vi "Write Packet Buffer.vi"(0 "data fifo in":refnum<k21>, 1 "reset":bool, 5 "sizes fifo in":refnum<k21>, 7 "serialized data":u8[](array[numeric])=[0, 0, 0, 0, 0, 0, 0, 0], 9 "input valid":bool, 11 "valid bytes in":fxp<+,4,4>, 12 "end of packet":bool) -> (4 "data fifo out":refnum<k21>, 6 "sizes fifo out":refnum<k21>, 14 "ready for input":bool)   [LabVIEW 2020, in "GettingStarted_Acq_Tap_148X_FPGA.lvlib"]
uses:
  <instrlib>/_niInstr/Data Formatting/v1/FPGA/Private/Convert/U8 array to Boolean Array.vi
  <vilib>/rvi/DataTransferAndStorage/Container/Common/niFpgaContainerExecOnDevCompGetState.vi
  <vilib>/rvi/Emulation/niFpgaEmulationIsFPGAContextNoSignature.vi
  <vilib>/rvi/Emulation/niFpgaSctlEmulationGetInTimedLoop.vi
  <vilib>/rvi/errors/niFpgaSetErrorForExecOnDevCompSimple.vi
  <vilib>/rvi/eio/common/nirviEmuReportErrorAndStop.vi
  <vilib>/rvi/DataTransferAndStorage/Container/Common/niFpgaContainerGetUniqueNameForEmu.vi
  <vilib>/rvi/FIFO/Fifo_Resource/nirvififoEmulationSetSize.vi
  <vilib>/rvi/FIFO/Fifo_Resource/nirviFifoEmulationQueueMgr.vi
  <instcachedir>/0/nirviFifoEmulationQueueMgr_E5CAEC123FF24DC58D834DCA3CDAA9B5.lvgen/nirviFifoEmulationQueueMgr_E5CAEC123FF24DC58D834DCA3CDAA9B5_000.vi
  <vilib>/rvi/FIFO/Fifo_Resource/nirvififoEmulationDetermineInputValidOut.vi
  <vilib>/rvi/FIFO/Fifo_Resource/nirvififoEmulationCreateLock.vi
  <vilib>/rvi/Emulation/niFpgaProcessEmulError.vi
  <vilib>/rvi/FIFO/Fifo_Resource/nirvififoEmulationObtainLock.vi
  <vilib>/rvi/FIFO/Fifo_Resource/nirvififoEmulationReleaseLock.vi
  <vilib>/rvi/occurrence/nirviWaitOnOccurrenceBase.vi
  <vilib>/rvi/errors/nirviReportUnexpectedCaseInternalError.vi
  <vilib>/rvi/errors/nirviReportUnexpectedCaseInternalError (U32).vi
  <vilib>/Utility/error.llb/Clear Errors.vi
  <vilib>/rvi/interface/RandomDataEmulation/niFpgaRandomDataHandleErrors.vi
  <instcachedir>/0/nirviFifoEmulationQueueMgr_E5CAEC123FF24DC58D834DCA3CDAA9B5.lvgen/nirviFifoEmulationQueueMgr_E5CAEC123FF24DC58D834DCA3CDAA9B5_012.vi
  <vilib>/rvi/DataTransferAndStorage/Container/XNode/niFpgaContainer.xnode
  <vilib>/rvi/FIFO/Fifo_Resource/niFpgaFifoEmulationRefIn.vi
  GettingStarted_Acq_Tap_148X_FPGA.lvlib
  <instrlib>/_niInstr/Data Formatting/v1/FPGA/niInstr Data Formatting v1 FPGA.lvlib
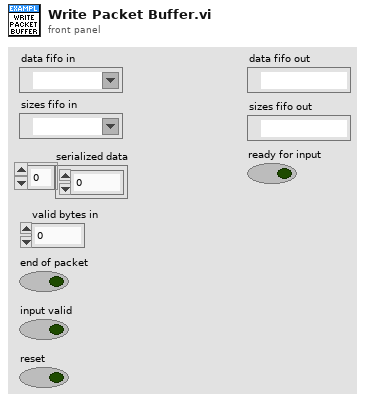
[diagram p1: front panel]
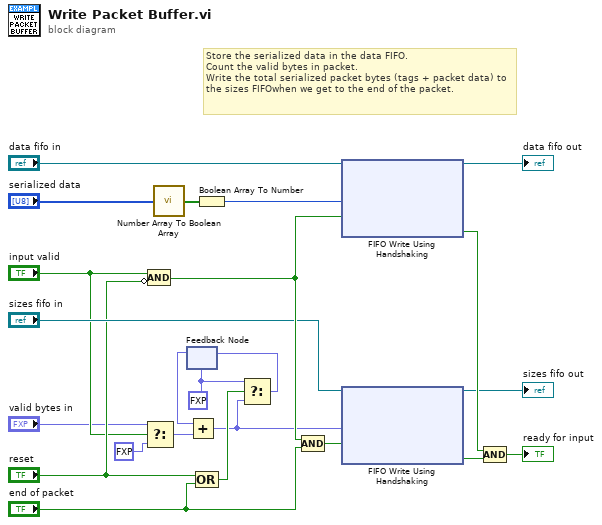
[diagram p0: block diagram]
diagram:
  w13 = fxp<+,17,17> 0.0 ("valid bytes in")
  # "Store the serialized data in the data FIFO.\nCount the valid bytes in packet.\nWrite the total serialized packet bytes (tags + packet data) to the sizes FIFOwhen we get to the end of the packet."
  n1 = Select(t="valid bytes in", s="input valid", f=fxp<+,4,4> 0.0) -> (s? t:f=w2:fxp<+,4,4>)
  n2 = Compound Arithmetic op=AND("input valid", invert "reset") -> (w20:bool)
  n3 = call-poly <instrlib>:"Number Array To Boolean Array.vi"("data in"="serialized data") -> ("data out"=w10:bool[])  [unwired: 14 in]
  n4 = feedback #1(w13) -> (w4:fxp<+,17,17>)
  n5 = Add(x=w4, y=w2) -> (x+y=w16:fxp<+,17,17>)
  n6 = Compound Arithmetic op=OR("reset", "end of packet") -> (w19:bool)
  n7 = Boolean Array To Number(Boolean array=w10) -> (number=w12:u64)
  n8 = Select(t=w13, s=w19, f=w16) -> (s? t:f=w14:fxp<+,17,17>)
  n9 = feedback-in #1(w14) -> ()
  n10 = Compound Arithmetic op=AND(w20, "end of packet") -> (w17:bool)
  n11 = xnode ("FIFO Write Using Handshaking")("Element"=w12, "Input Valid"=w20, "FIFO In"="data fifo in") -> ("Ready for Input"=w21:bool, "FIFO Out"=→"data fifo out":refnum<k21>)
  n12 = xnode ("FIFO Write Using Handshaking")("Element"=w16, "Input Valid"=w17, "FIFO In"="sizes fifo in") -> ("Ready for Input"=w22:bool, "FIFO Out"=→"sizes fifo out":refnum<k21>)
  n13 = Compound Arithmetic op=AND(w21, w22) -> (→"ready for input":bool)
